vi "Read Queued Processed Outgoing Messages.vi"(8 "error in (no error)":errorcluster, 11 "J1939 Cluster":T2) -> (0 "error out":errorcluster, 2 "timed out?":bool, 3 "Frames":T1[](array[typedef]) {"Identifier" format="%08x"})   [LabVIEW 2013, in "J1939 Addon Engine.lvlib"]
uses:
  Engine/J1939 Addon Engine.lvlib
  Types/Setup Information Cluster.ctl
  <vilib>/xnet/xnet.llb/XNET Frame CAN.ctl
  <vilib>/xnet/xnet.llb/XNET Frame Type CAN.ctl
  J1939 Utilities/Types/CAN Outgoing Message Cluster.ctl
  J1939 Utilities/J1939 Utilities.lvlib
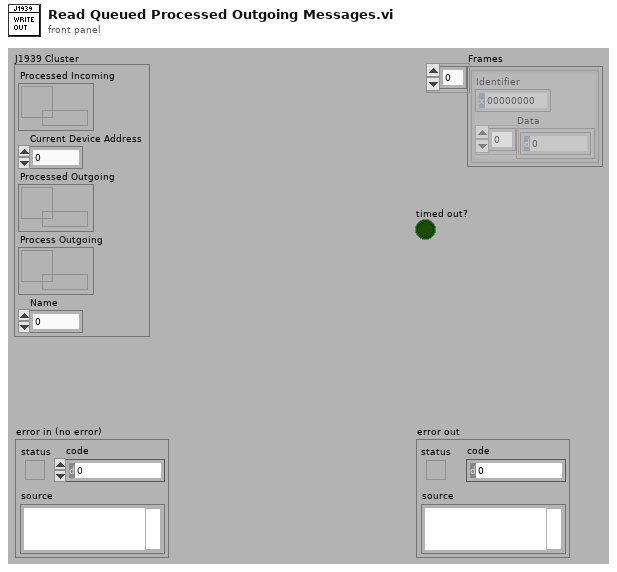
[diagram p1: front panel]
types:
  T1 = typedef "J1939 Addon Shared.lvlib/J1939 Utilities.lvlib/CAN Outgoing Message Cluster.ctl" = cluster{"Identifier":u32, "Data":u8[]}
  T2 = typedef "J1939 Addon Engine.lvlib/Setup Information Cluster.ctl" = cluster{"Processed Incoming":refnum<queue>, "Current Device Address":u8, "Processed Outgoing":refnum<queue>, "Process Outgoing":refnum<queue>, "Name":u64}
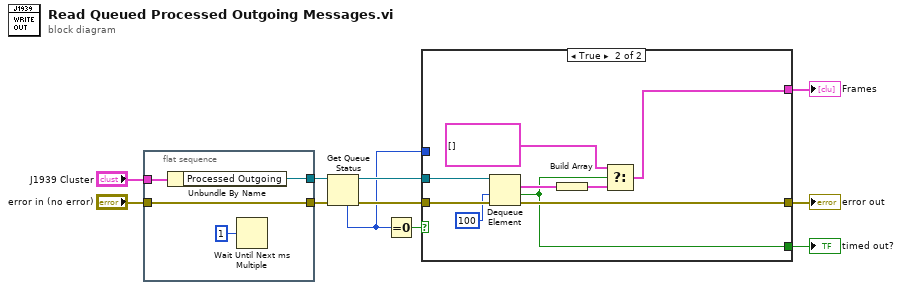
[diagram p0: block diagram]
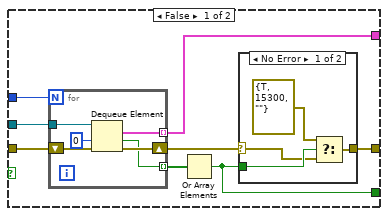
[diagram p2: hidden frame]
diagram:
  n1 = flat-sequence {
    tunnel: [w15] -> w7
    tunnel: "J1939 Cluster" -> [w14]
    tunnel: [w12] -> w2
    tunnel: "error in (no error)" -> [w12]
    frame #0 {
      n2 = Unbundle By Name(w14) -> ("Processed Outgoing"=w15:refnum<queue>)
      n3 = Wait Until Next ms Multiple(millisecond multiple=u32 1) -> ()  [unwired: 1 out]
    }
  }
  n4 = Get Queue Status(queue=w7, error in (no error)=w2) -> (queue out=w11:refnum<queue>, error out=w10:errorcluster, # elements in queue=w8:i32)  [unwired: 6 out]
  n5 = Equal To 0?(x=w8) -> (x = 0?=w9:bool)
  n6 = case shown="True" w9 {
    tunnel: [w17 w40] -> w4
    tunnel: w11 -> [w23 w43]
    tunnel: w10 -> [w21 w42]
    tunnel: [w22 w37] -> w5
    tunnel: w8 -> [w20 _]
    tunnel: [w18 w35] -> w3
    frame False {
      n7 = for {
        N: w20 -> [_]
        tunnel: w23 -> [w33]
        tunnel: [w32] -> w22 mode=indexing
        shift-right: [w34] -> w16
        shift-left: w21 -> [w31]
        tunnel: [w30] -> w19 mode=indexing
        n8 = Dequeue Element(queue=w33, timeout in ms (-1)=0, error in (no error)=w31) -> (element=w32:T1, timed out?=w30:bool, error out=w34:errorcluster)  [unwired: 1 out]
      }
      n9 = Or Array Elements(Boolean array=w19) -> (logical OR=w18:bool)
      n10 = case shown="No Error" w16 {
        selector: w16 -> [w24 w28]
        tunnel: w18 -> [w27 _]
        tunnel: [w26 w28] -> w17
        frame No Error {
          n11 = Select(t=errorcluster {"status"=TRUE, "code"=15300, "source"=""}, s=w27, f=w24) -> (s? t:f=w26:errorcluster)
        }
        frame Error {
        }
      }
    }
    frame True {
      n12 = Dequeue Element(queue=w43, timeout in ms (-1)=100, error in (no error)=w42) -> (element=w39:T1, timed out?=w35:bool, error out=w40:errorcluster)  [unwired: 1 out]
      n13 = Build Array(w39) -> (w38:T1[])
      n14 = Select(t=T1[] [], s=w35, f=w38) -> (s? t:f=w37:T1[])
    }
  }
  "Frames" <- w5
  "error out" <- w4
  "timed out?" <- w3
